vi "GetFile.vi"(8 "name":string, 9 "HighSpeedEServer":refnum<k24>, 11 "error in (no error)":errorcluster) -> (1 "Content":string, 3 "error out":errorcluster)   [LabVIEW 2024, in "UnderAutomation.Yaskawa.lvlib"]
uses:
  UnderAutomation.Yaskawa.lvlib
  C:/Users/fg/Documents/Yaskawa.vi/LabVIEW_2024/UnderAutomation.Yaskawa/lib/UnderAutomation.Yaskawa.dll
  lib/UnderAutomation.Yaskawa.dll
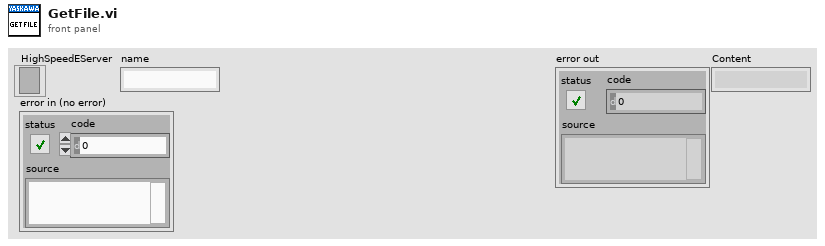
[diagram p1: front panel]
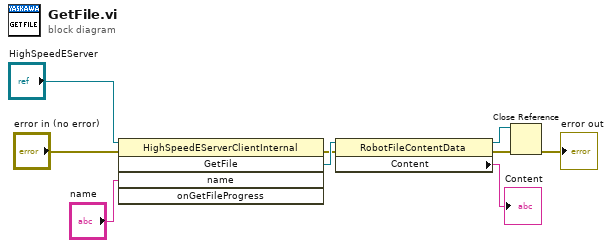
[diagram p0: block diagram]
diagram:
  n1 = invoke class="HighSpeedEServerClientInternal" method="GetFile"(reference="HighSpeedEServer", error in="error in (no error)", "name"="name") -> (error out=w5:errorcluster, "GetFile"=w6:refnum<k24>)  [unwired: 2 in, 3 out]
  n2 = property class="RobotFileContentData"(reference=w6, error in=w5) -> (reference out=w1:refnum<k24>, error out=w3:errorcluster, "Content"=→"Content":string)
  n3 = Close Reference(reference=w1, error in (no error)=w3) -> (error out=→"error out":errorcluster)
